vi "Initialize.vi"(8 "error in (no error)":errorcluster caption="错误输入（无错误）", 10 "VISA资源名称":refnum<visa-resource-name>, 11 "Fluke 8808A 输入":refnum<class "Fluke 8808A.lvclass">) -> (0 "error out":errorcluster caption="错误输出", 3 "Fluke 8808A 输出":refnum<class "Fluke 8808A.lvclass">)   [LabVIEW 2020, in "Fluke 8808A.lvlib" / "Fluke 8808A.lvclass"]
uses:
  Fluke 8808A.lvclass
  <instrlib>/Fluke 8808/Fluke 8808.lvlib
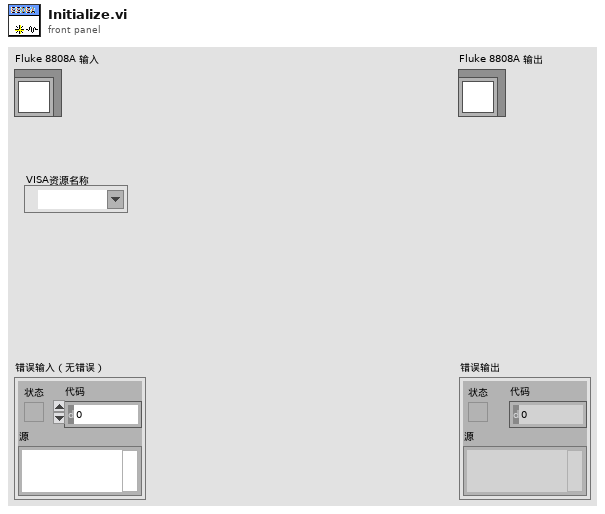
[diagram p1: front panel]
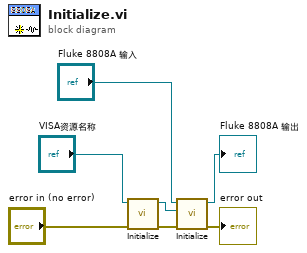
[diagram p0: block diagram]
diagram:
  n1 = call <instrlib>:"Initialize.vi"("error in (no error)"="error in (no error)", "VISA resource name"="VISA资源名称") -> ("error out"=w1:errorcluster, "VISA resource name out"=w6:refnum<visa-resource-name>)  [unwired: 8 in]
  n2 = call-parent <instrlib>:"Initialize.vi"("error in (no error)"=w1, "VISA资源名称"=w6, "数字多用表接口 输入"="Fluke 8808A 输入") -> ("error out"=→"error out":errorcluster, "数字多用表接口 输出"=→"Fluke 8808A 输出":refnum<class "Fluke 8808A.lvclass">)  [unwired: 7 in]
